vi "ep_Check Synchronous Speed.vi"(8 "error in (no error)":errorcluster, 10 "synchronous speed [RPM]":dbl, 11 "nominal frequency":enum16{"50 Hz", "60 Hz"}(ring)) -> (0 "error out":errorcluster)   [LabVIEW 2014, in "NI_EP_Motor Monitoring.lvlib"]
uses:
  <vilib>/addons/Electrical Power/Motor Monitoring/NI_EP_Motor Monitoring.lvlib
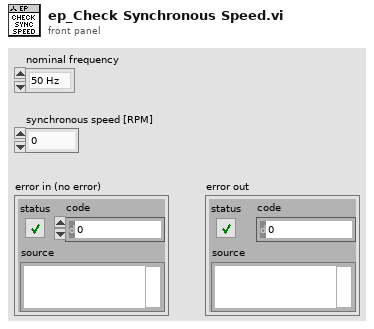
[diagram p1: front panel]
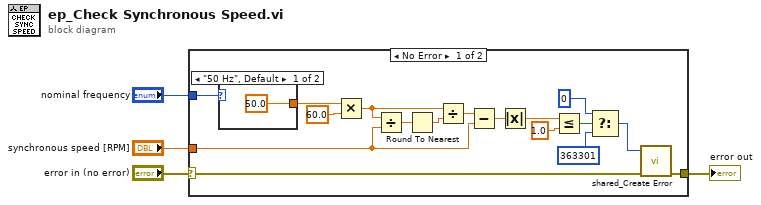
[diagram p0: block diagram]
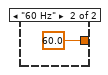
[diagram p2: hidden frame]
diagram:
  n1 = case shown="No Error" "error in (no error)" {
    selector: "error in (no error)" -> [w5 w24]
    tunnel: "nominal frequency" -> [w8 _]
    tunnel: "synchronous speed [RPM]" -> [w7 _]
    tunnel: [w6 w24] -> w1
    frame No Error {
      n2 = case shown="\"50 Hz\", Default" w8 {
        tunnel: [50.0 60.0] -> w10
        frame "50 Hz", Default {
        }
        frame "60 Hz" {
        }
      }
      n3 = Multiply(x=w10, y=60.0) -> (x*y=w9:dbl)
      n4 = Divide(x=w9, y=w7) -> (x/y=w20:dbl)
      n5 = Round To Nearest(number=w20) -> (nearest integer value=w19:dbl)
      n6 = Divide(x=w9, y=w19) -> (x/y=w18:dbl)
      n7 = Subtract(x=w18, y=w7) -> (x-y=w17:dbl)
      n8 = Absolute Value(x=w17) -> (abs(x)=w16:dbl)
      n9 = Less Or Equal?(x=w16, y=1.0) -> (x <= y?=w14:bool)
      n10 = Select(t=0 ("y"), s=w14, f=363301 ("y")) -> (s? t:f=w12:i32)
      n11 = call <vilib>:"shared_Create Error.vi"("error in (no error)"=w5, "error code (0)"=w12) -> ("error out"=w6:errorcluster)  [unwired: 9 in]
    }
    frame Error {
    }
  }
  "error out" <- w1
